vi "AlGaInPAs_v20c.vi"(2 "Debug Mode":bool, 3 "Elapsed Time(s)":dbl, 4 "State":enum16{"Edit", "Start", "Run", "End", "Idle"}(ring), 5 "Argument List In":string[](array[string])) -> (0 "Status Out":string, 1 "Argument List Out":string[](array[string]))   [LabVIEW 2011]
uses:
  high_level_proc/source_noDilute.ctl
  high_level_proc/source_noDilution.ctl
panel:
  in  "Array":refnum<vi>[](array[refnum])
  in  "Al bubbler":T1 caption="Al" {"Flow" format="%.2f"}
  in  "Se bubbler":T2={"Dilution"=FALSE, "Calculated"=0, "MFC1 flow"=0.0, "MFC2 flow"=10.0, "MFC3 flow"=100.0, "Bubbler (main)"={"Flow"=0.0, "Prep"=FALSE, "Run"=FALSE, "Active"=FALSE}} caption="Al" {"Bubbler (main)"."Flow" format="%.2f"; "MFC1 flow" format="%.4f"; "MFC3 flow" format="%.1f"; "MFC2 flow" format="%.2f"; "Calculated" items=["Flow", "MFC1", "MFC2", "MFC3"]}
  in  "P bubbler":T1 caption="Al" {"Flow" format="%.2f"}
  in  "As gas":T1 caption="Al" {"Flow" format="%.2f"}
  in  "P gas":T1 caption="Al" {"Flow" format="%.2f"}
  in  "In bubbler":T1 caption="Al" {"Flow" format="%.2f"}
  in  "Tab Control":T3(tab)
  out "Al Prep":bool caption="Pre-run"
  out "Al Run":bool caption="Run"
  out "Al Flow":dbl caption="Al Flow (0-100 sscm)" format="%.2f"
  out "Ga MFC1 flow":dbl caption="R1 (0-10 sscm)" format="%.4f"
  out "Ga MFC3 flow":dbl=100.0 caption="R3 (0-1000 sscm)" format="%.1f"
  out "Ga MFC2 flow":dbl=10.0 caption="R2 (0-100 sscm)" format="%.2f"
  out "Ga Calculated":u16(ring)=1 caption="Calculated" items=["Ga flow", "MFC1", "MFC2", "MFC3"]
  out "Ga Dilution":bool caption="Dilute"
  out "Ga Prep":bool caption="Pre-run"
  out "Ga Run":bool caption="Run"
  out "Ga Flow":dbl caption="Ga Flow (0-10 sscm)" format="%.2f"
  out "In Prep":bool caption="Pre-run"
  out "In Run":bool caption="Run"
  out "In Flow":dbl caption="In Flow (0-100 sscm)" format="%.2f"
  out "P gas Run":bool caption="Run"
  out "P gas Prep":bool caption="Pre-run"
  out "P gas Flow":dbl caption="PH3 Flow (0-100 sscm)" format="%.2f"
  out "As gas Prep":bool caption="Pre-run"
  out "As gas Run":bool caption="Run"
  out "As gas Flow":dbl caption="AsH3 Flow (0-10 sscm)" format="%.2f"
  out "P liq Prep":bool caption="Pre-run"
  out "P liq Run":bool caption="Run"
  out "P liq Flow":dbl caption="P bubbler Flow (0-100 sscm)" format="%.2f"
  out "Se MFC1 flow":dbl caption="R1 (0-10 sscm)" format="%.4f"
  out "Se MFC3 flow":dbl=100.0 caption="R3 (0-1000 sscm)" format="%.1f"
  out "Se MFC2 flow":dbl=10.0 caption="R2 (0-100 sscm)" format="%.2f"
  out "Se Calculated":u16(ring)=1 caption="Calculated" items=["Ga flow", "MFC1", "MFC2", "MFC3"]
  out "Se Dilution":bool caption="Dilute"
  out "Se Prep":bool caption="Pre-run"
  out "Se Run":bool caption="Run"
  out "Se Flow":dbl caption="Se Flow (0-10 sscm)" format="%.2f"
  in  "Ga bubbler":T2={"Dilution"=FALSE, "Calculated"=0, "MFC1 flow"=0.0, "MFC2 flow"=10.0, "MFC3 flow"=100.0, "Bubbler (main)"={"Flow"=0.0, "Prep"=FALSE, "Run"=FALSE, "Active"=FALSE}} caption="Al" {"Bubbler (main)"."Flow" format="%.2f"; "MFC1 flow" format="%.4f"; "MFC3 flow" format="%.1f"; "MFC2 flow" format="%.2f"; "Calculated" items=["Flow", "MFC1", "MFC2", "MFC3"]}
  out "prep_done":bool
  out "run started":bool
  out "first":bool=TRUE
  out "total time":dbl
  out "is OK?":bool
  in  "prep_time":dbl
  in  "Cancel":bool
  in  "OK":bool
  out "tTotal(s) 2":dbl
  # "s"
  # "Add pre-run time to run time in editor."
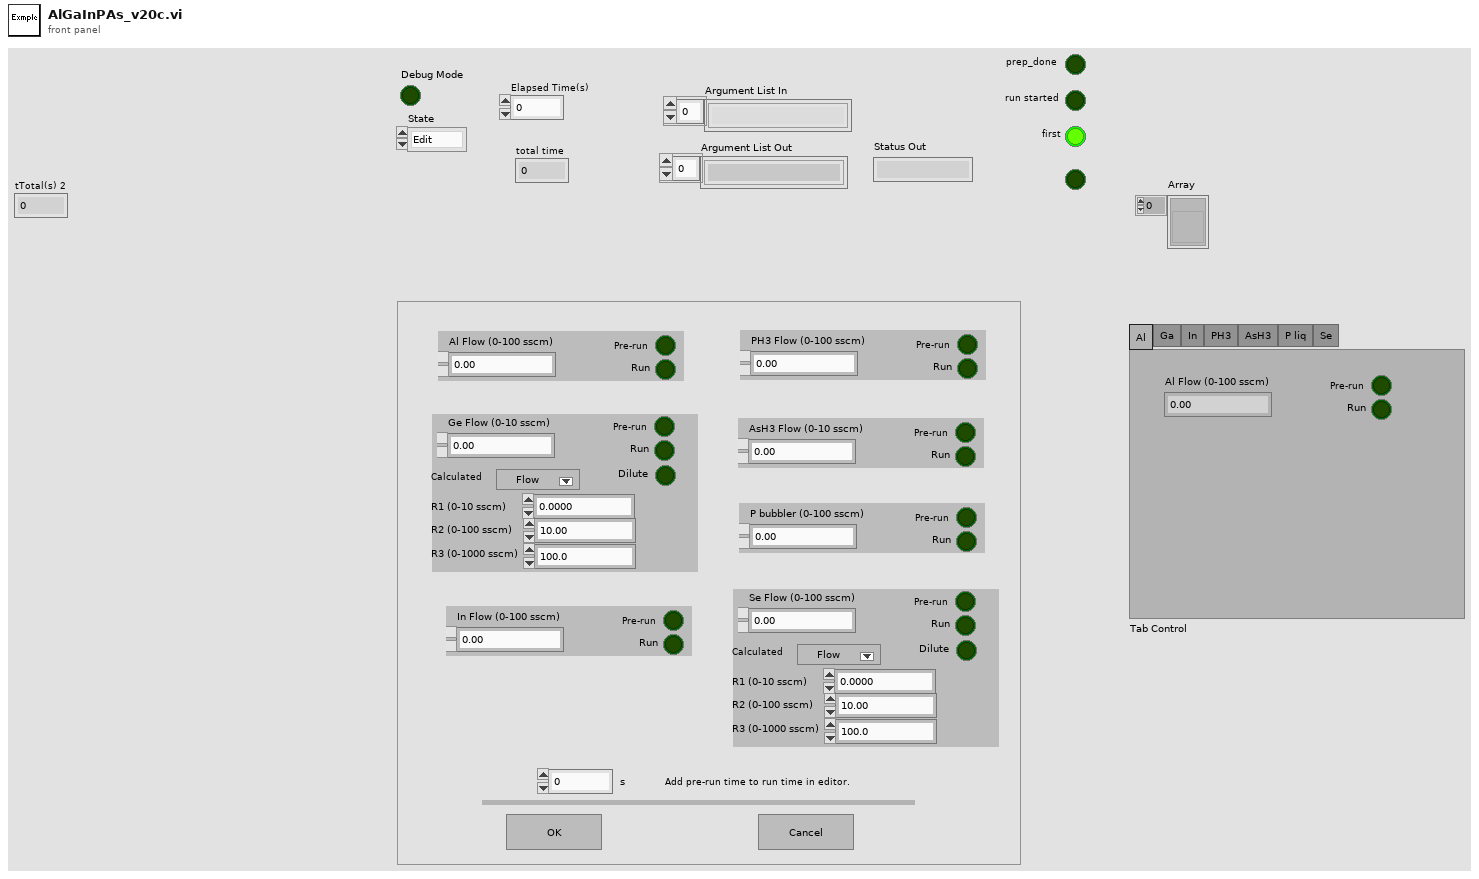
[diagram p1: front panel]
types:
  T1 = typedef "source_noDilution.ctl" = cluster{"Flow":dbl, "Prep":bool, "Run":bool, "Active":bool}
  T2 = typedef "source_noDilute.ctl" = cluster{"Dilution":bool, "Calculated":u16, "MFC1 flow":dbl, "MFC2 flow":dbl, "MFC3 flow":dbl, "Bubbler (main)":T1}
  T3 = enum32{"Al", "Ga", "In", "PH3", "AsH3", "P liq", "Se"}
  T4 = enum16{"Discrete", "Continuous", "Instantaneous", "Finite"}
  T5 = enum32{"Invalid", "Default", "Floating", "Floating/Auto-Hide", "Modal"}
  T6 = enum8{"Enabled", "Disabled", "Disabled and Grayed Out"}
  T7 = cluster{"Flow":dbl, "Prep":bool, "Run":bool, "Active":bool}
  T8 = cluster{"Dilution":bool, "Calculated":u16, "MFC1 flow":dbl, "MFC2 flow":dbl, "MFC3 flow":dbl, "Bubbler (main)":T1}
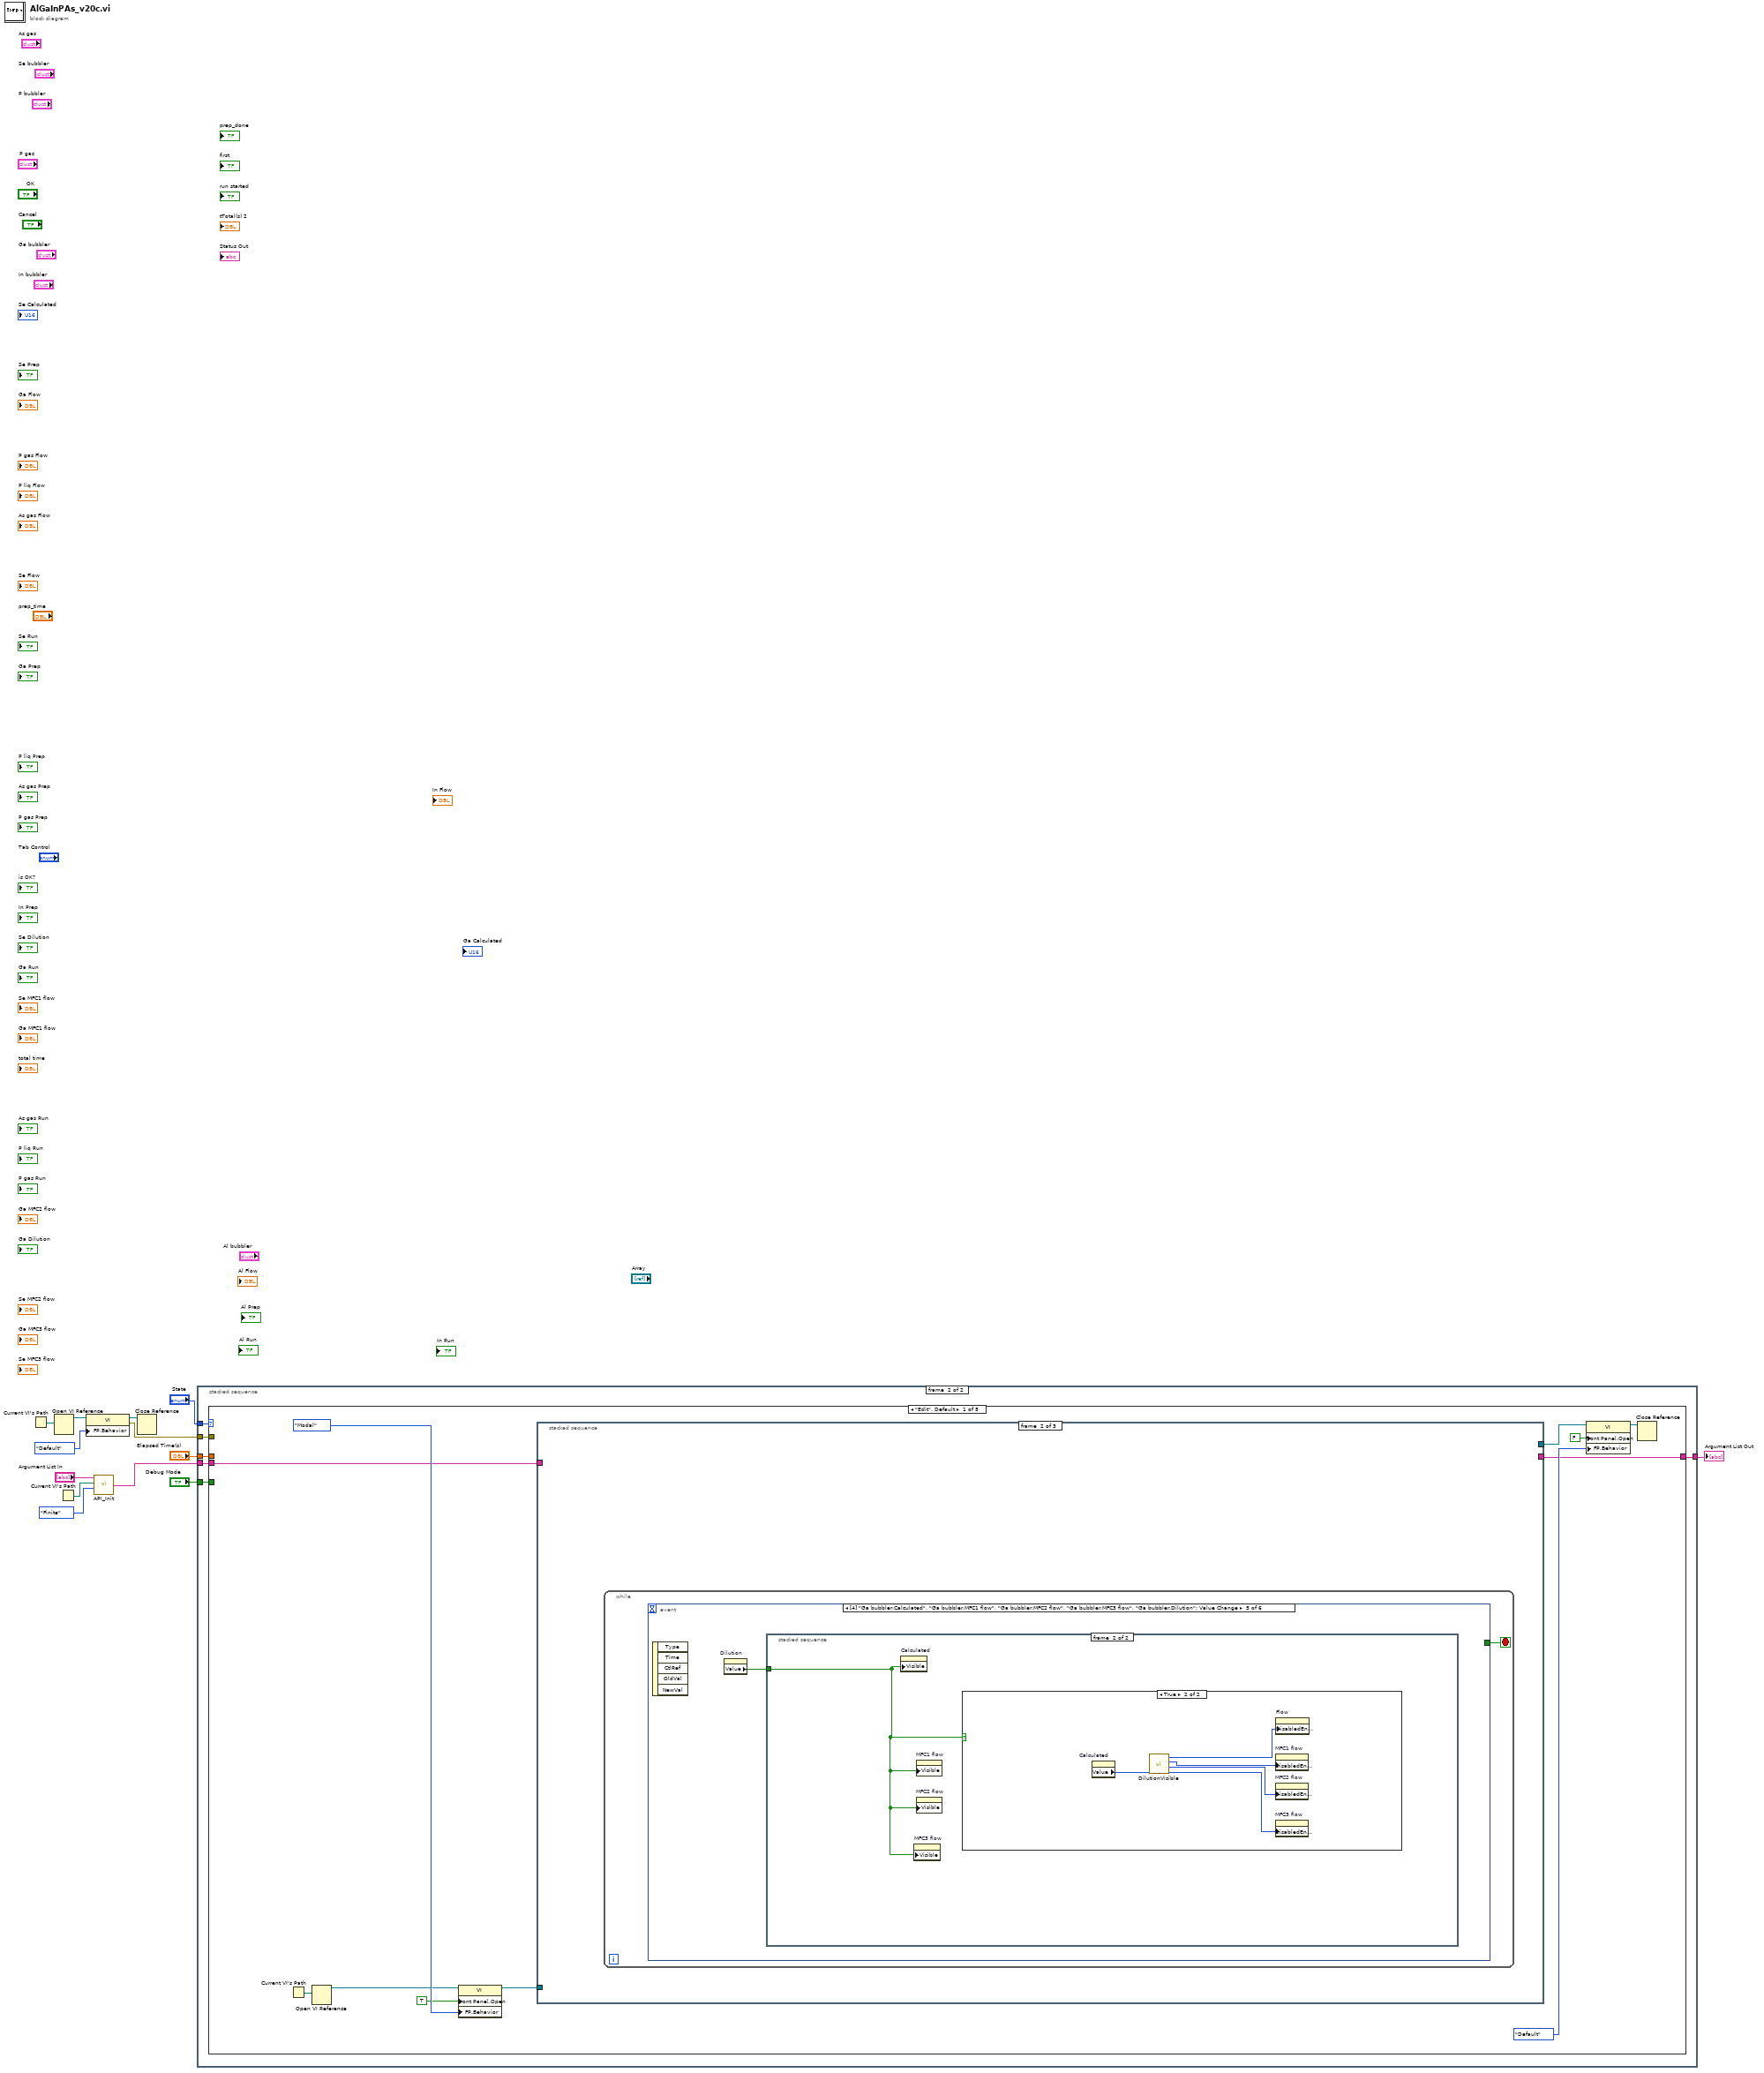
[diagram p0: block diagram]
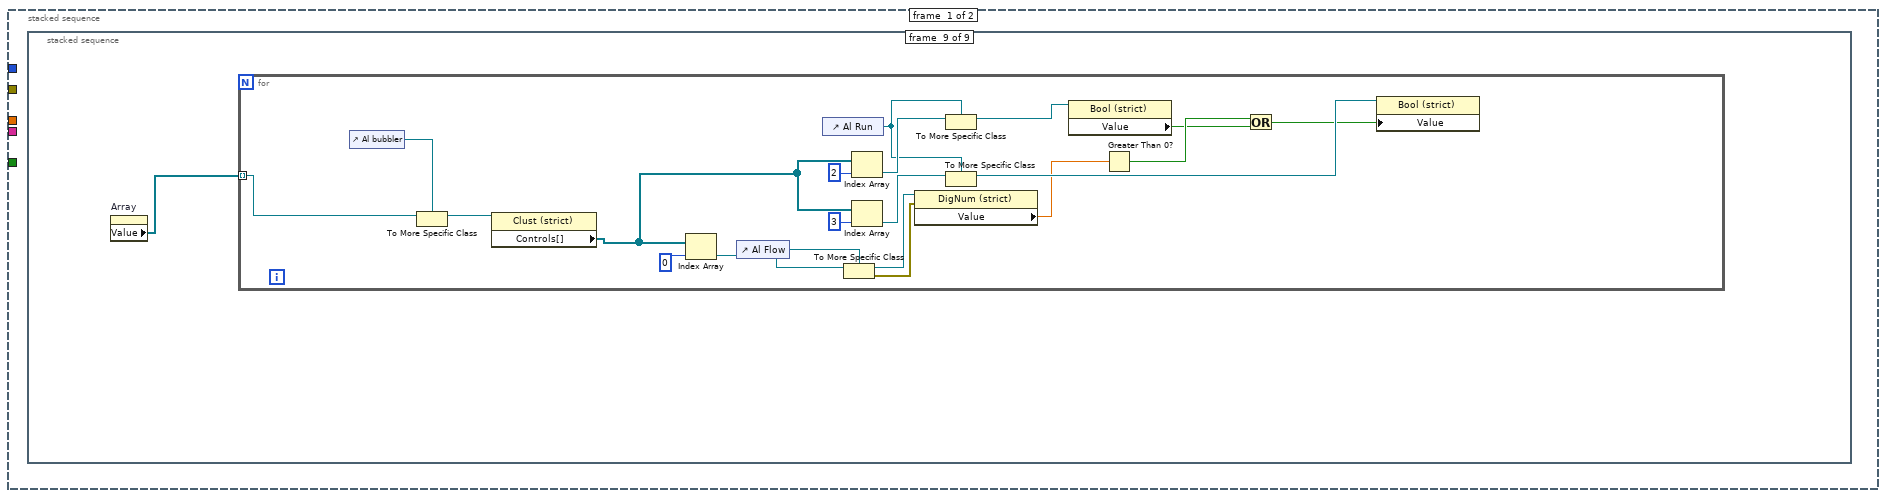
[diagram p2: hidden frame]
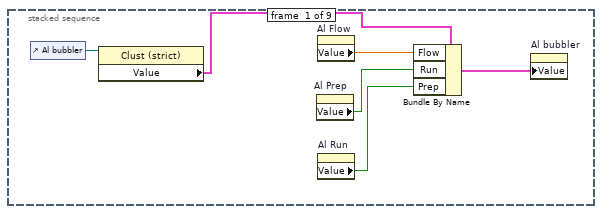
[diagram p3: hidden frame]
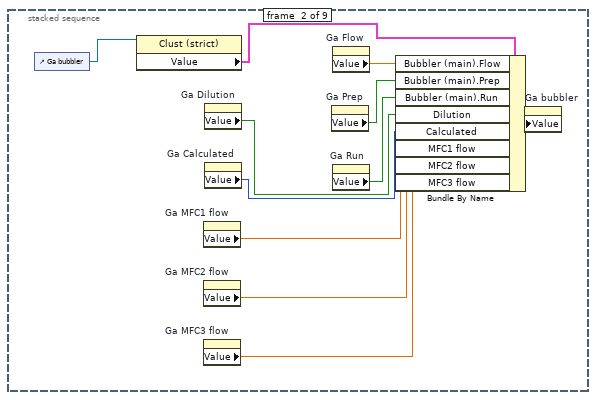
[diagram p4: hidden frame]
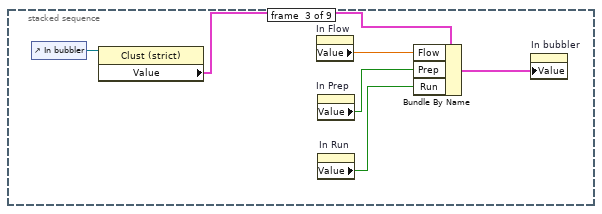
[diagram p5: hidden frame]
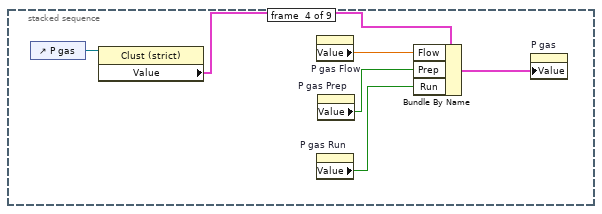
[diagram p6: hidden frame]
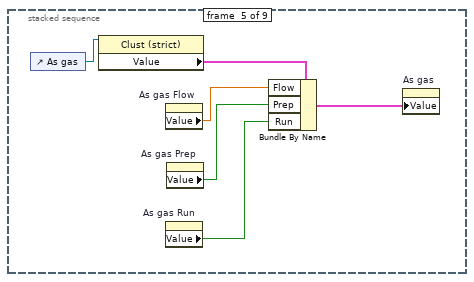
[diagram p7: hidden frame]
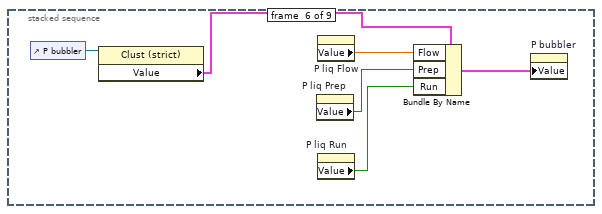
[diagram p8: hidden frame]
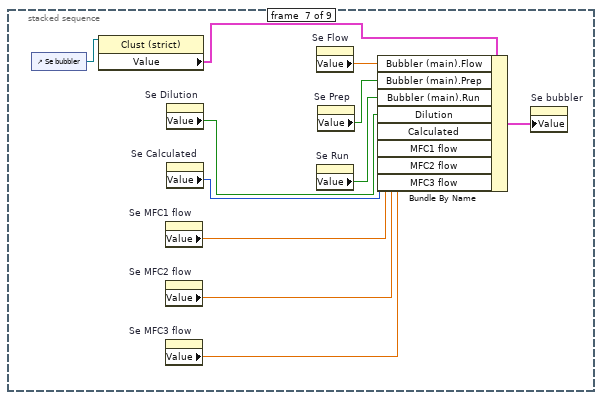
[diagram p9: hidden frame]
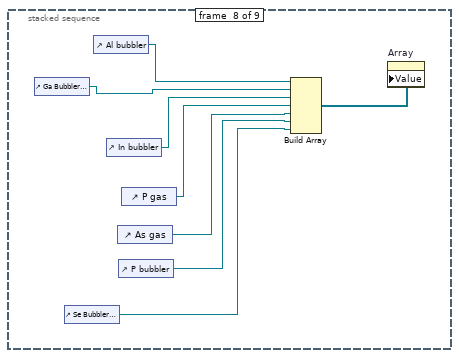
[diagram p10: hidden frame]
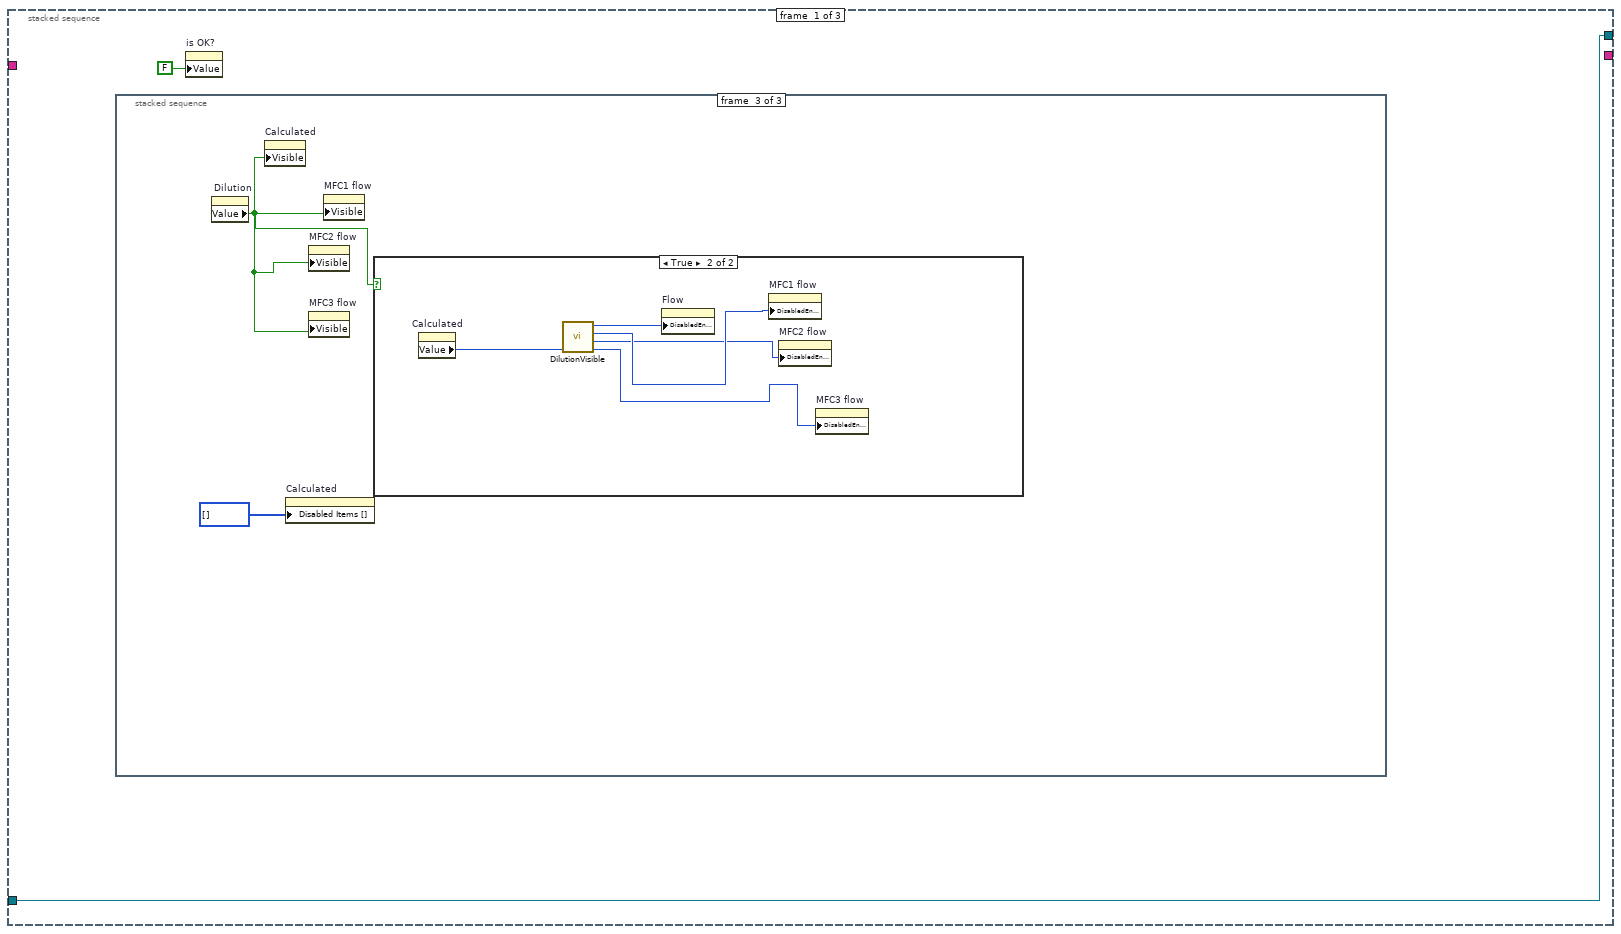
[diagram p11: hidden frame]
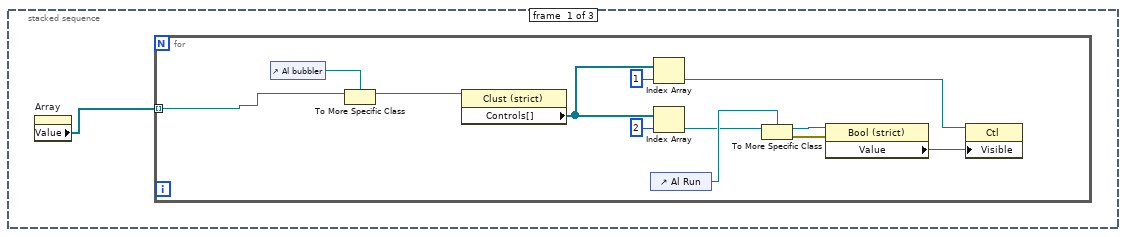
[diagram p12: hidden frame]
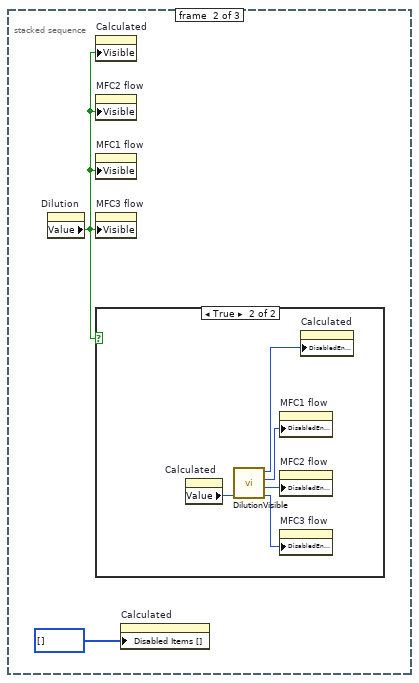
[diagram p13: hidden frame]
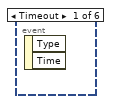
[diagram p16: hidden frame]
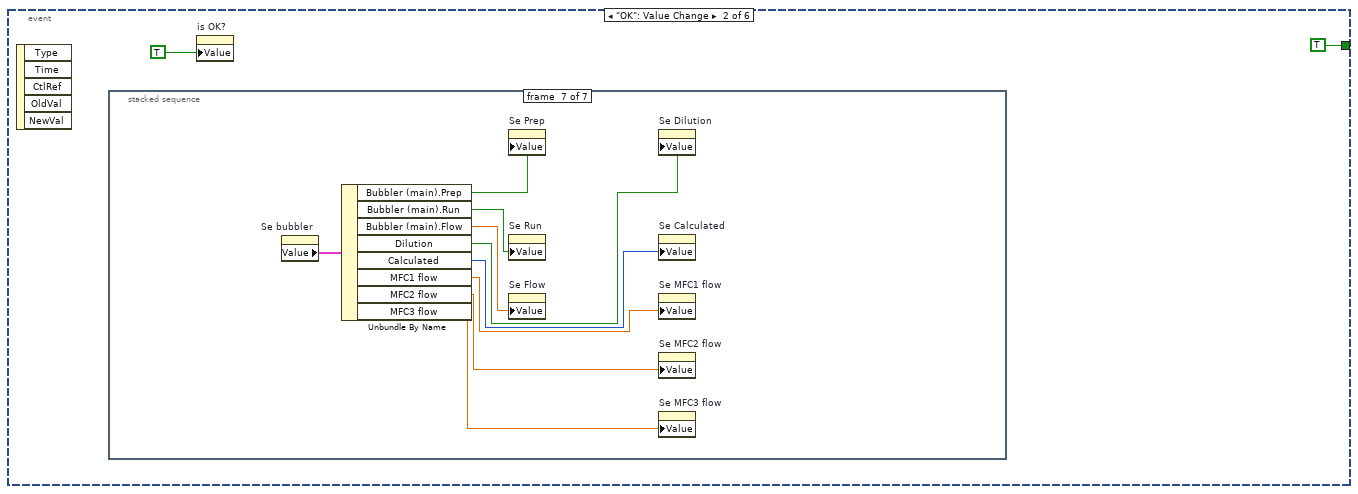
[diagram p17: hidden frame]
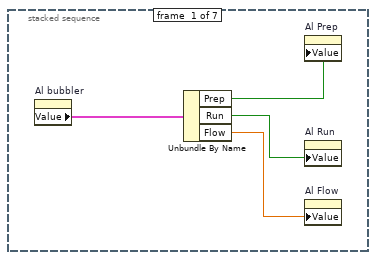
[diagram p18: hidden frame]
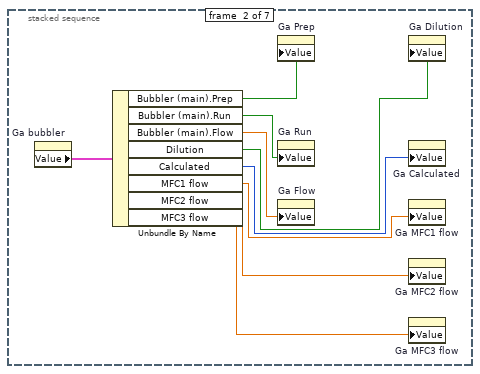
[diagram p19: hidden frame]
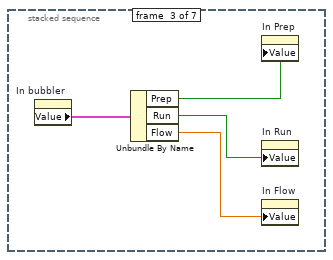
[diagram p20: hidden frame]
diagram:
  n1 = Current VI's Path() -> (path=w9:path)
  n2 = Open VI Reference(vi path=w9) -> (vi reference=w8:refnum<vi>)  [unwired: 1 in, 5 out]
  n3 = Current VI's Path() -> (path=w4:path)
  n4 = property class="VI"(reference=w8, "FP.Behavior"=T5."Default" ("Front Panel Window:Behavior")) -> (reference out=w6:refnum<vi>, error out=w5:errorcluster)  [unwired: 1 in]
  n5 = call "API_Init.vi"("API Mode"=T4."Finite", "VI Path"=w4, "Argument List In"="Argument List In") -> ("Argument List Out"=w1:string[])  [unwired: 1 in]
  n6 = Close Reference(reference=w6) -> ()  [unwired: 1 in, 1 out]
  n7 = stacked-sequence {
    tunnel: "State" -> [_ w100]
    tunnel: "Debug Mode" -> [_ w99]
    tunnel: "Elapsed Time(s)" -> [_ w98]
    tunnel: [_ w97] -> w10
    tunnel: w5 -> [_ w96]
    tunnel: w1 -> [_ w95]
    frame #0 {
      n8 = stacked-sequence {
        frame #0 {
          n9 = control-ref of="Al bubbler"() -> (w16:refnum<vi>)
          n10 = property class="Clust (strict)"(reference=w16) -> ("Value"=w15:T7)  [unwired: 1 in, 2 out]
          n11 = property on="Al Prep" class="Bool (strict)"() -> ("Value"=w18:bool)  [unwired: 2 in, 2 out]
          n12 = property on="Al Flow" class="DigNum (strict)"() -> ("Value"=w19:dbl)  [unwired: 2 in, 2 out]
          n13 = property on="Al Run" class="Bool (strict)"() -> ("Value"=w17:bool)  [unwired: 2 in, 2 out]
          n14 = Bundle By Name(cluster=w15, "Flow"=w19, "Run"=w18, "Prep"=w17) -> (w14:T7)
          n15 = property on="Al bubbler" class="Clust (strict)"("Value"=w14) -> ()  [unwired: 2 in, 2 out]
        }
        frame #1 {
          n16 = control-ref of="Ga bubbler"() -> (w20:refnum<vi>)
          n17 = property class="Clust (strict)"(reference=w20) -> ("Value"=w21:T8)  [unwired: 1 in, 2 out]
          n18 = property on="Ga MFC1 flow" class="DigNum (strict)"() -> ("Value"=w28:dbl)  [unwired: 2 in, 2 out]
          n19 = property on="Ga MFC2 flow" class="DigNum (strict)"() -> ("Value"=w29:dbl)  [unwired: 2 in, 2 out]
          n20 = property on="Ga MFC3 flow" class="DigNum (strict)"() -> ("Value"=w30:dbl)  [unwired: 2 in, 2 out]
          n21 = property on="Ga Dilution" class="Bool (strict)"() -> ("Value"=w27:bool)  [unwired: 2 in, 2 out]
          n22 = property on="Ga Calculated" class="Ring (strict)"() -> ("Value"=w25:u16)  [unwired: 2 in, 2 out]
          n23 = property on="Ga Prep" class="Bool (strict)"() -> ("Value"=w24:bool)  [unwired: 2 in, 2 out]
          n24 = property on="Ga Flow" class="DigNum (strict)"() -> ("Value"=w23:dbl)  [unwired: 2 in, 2 out]
          n25 = property on="Ga Run" class="Bool (strict)"() -> ("Value"=w26:bool)  [unwired: 2 in, 2 out]
          n26 = Bundle By Name(cluster=w21, "Bubbler (main).Flow"=w23, "Bubbler (main).Prep"=w24, "Bubbler (main).Run"=w26, "Dilution"=w27, "Calculated"=w25, "MFC1 flow"=w28, "MFC2 flow"=w29, "MFC3 flow"=w30) -> (w22:T8)
          n27 = property on="Ga bubbler" class="Clust (strict)"("Value"=w22) -> ()  [unwired: 2 in, 2 out]
        }
        frame #2 {
          n28 = control-ref of="In bubbler"() -> (w31:refnum<vi>)
          n29 = property class="Clust (strict)"(reference=w31) -> ("Value"=w32:T7)  [unwired: 1 in, 2 out]
          n30 = property on="In Flow" class="DigNum (strict)"() -> ("Value"=w33:dbl)  [unwired: 2 in, 2 out]
          n31 = property on="In Prep" class="Bool (strict)"() -> ("Value"=w35:bool)  [unwired: 2 in, 2 out]
          n32 = property on="In Run" class="Bool (strict)"() -> ("Value"=w36:bool)  [unwired: 2 in, 2 out]
          n33 = Bundle By Name(cluster=w32, "Flow"=w33, "Prep"=w35, "Run"=w36) -> (w34:T7)
          n34 = property on="In bubbler" class="Clust (strict)"("Value"=w34) -> ()  [unwired: 2 in, 2 out]
        }
        frame #3 {
          n35 = control-ref of="P gas"() -> (w37:refnum<vi>)
          n36 = property class="Clust (strict)"(reference=w37) -> ("Value"=w38:T7)  [unwired: 1 in, 2 out]
          n37 = property on="P gas Flow" class="DigNum (strict)"() -> ("Value"=w39:dbl)  [unwired: 2 in, 2 out]
          n38 = property on="P gas Run" class="Bool (strict)"() -> ("Value"=w42:bool)  [unwired: 2 in, 2 out]
          n39 = property on="P gas Prep" class="Bool (strict)"() -> ("Value"=w41:bool)  [unwired: 2 in, 2 out]
          n40 = Bundle By Name(cluster=w38, "Flow"=w39, "Prep"=w41, "Run"=w42) -> (w40:T7)
          n41 = property on="P gas" class="Clust (strict)"("Value"=w40) -> ()  [unwired: 2 in, 2 out]
        }
        frame #4 {
          n42 = control-ref of="As gas"() -> (w44:refnum<vi>)
          n43 = property class="Clust (strict)"(reference=w44) -> ("Value"=w43:T7)  [unwired: 1 in, 2 out]
          n44 = property on="As gas Flow" class="DigNum (strict)"() -> ("Value"=w46:dbl)  [unwired: 2 in, 2 out]
          n45 = property on="As gas Run" class="Bool (strict)"() -> ("Value"=w48:bool)  [unwired: 2 in, 2 out]
          n46 = property on="As gas Prep" class="Bool (strict)"() -> ("Value"=w47:bool)  [unwired: 2 in, 2 out]
          n47 = Bundle By Name(cluster=w43, "Flow"=w46, "Prep"=w47, "Run"=w48) -> (w45:T7)
          n48 = property on="As gas" class="Clust (strict)"("Value"=w45) -> ()  [unwired: 2 in, 2 out]
        }
        frame #5 {
          n49 = control-ref of="P bubbler"() -> (w49:refnum<vi>)
          n50 = property class="Clust (strict)"(reference=w49) -> ("Value"=w50:T7)  [unwired: 1 in, 2 out]
          n51 = property on="P liq Prep" class="Bool (strict)"() -> ("Value"=w53:bool)  [unwired: 2 in, 2 out]
          n52 = property on="P liq Flow" class="DigNum (strict)"() -> ("Value"=w52:dbl)  [unwired: 2 in, 2 out]
          n53 = property on="P liq Run" class="Bool (strict)"() -> ("Value"=w54:bool)  [unwired: 2 in, 2 out]
          n54 = Bundle By Name(cluster=w50, "Flow"=w52, "Prep"=w53, "Run"=w54) -> (w51:T7)
          n55 = property on="P bubbler" class="Clust (strict)"("Value"=w51) -> ()  [unwired: 2 in, 2 out]
        }
        frame #6 {
          n56 = control-ref of="Se bubbler"() -> (w55:refnum<vi>)
          n57 = property class="Clust (strict)"(reference=w55) -> ("Value"=w56:T8)  [unwired: 1 in, 2 out]
          n58 = property on="Se MFC1 flow" class="DigNum (strict)"() -> ("Value"=w63:dbl)  [unwired: 2 in, 2 out]
          n59 = property on="Se MFC2 flow" class="DigNum (strict)"() -> ("Value"=w64:dbl)  [unwired: 2 in, 2 out]
          n60 = property on="Se MFC3 flow" class="DigNum (strict)"() -> ("Value"=w65:dbl)  [unwired: 2 in, 2 out]
          n61 = property on="Se Dilution" class="Bool (strict)"() -> ("Value"=w61:bool)  [unwired: 2 in, 2 out]
          n62 = property on="Se Calculated" class="Ring (strict)"() -> ("Value"=w62:u16)  [unwired: 2 in, 2 out]
          n63 = property on="Se Flow" class="DigNum (strict)"() -> ("Value"=w58:dbl)  [unwired: 2 in, 2 out]
          n64 = property on="Se Run" class="Bool (strict)"() -> ("Value"=w60:bool)  [unwired: 2 in, 2 out]
          n65 = property on="Se Prep" class="Bool (strict)"() -> ("Value"=w59:bool)  [unwired: 2 in, 2 out]
          n66 = Bundle By Name(cluster=w56, "Bubbler (main).Flow"=w58, "Bubbler (main).Prep"=w59, "Bubbler (main).Run"=w60, "Dilution"=w61, "Calculated"=w62, "MFC1 flow"=w63, "MFC2 flow"=w64, "MFC3 flow"=w65) -> (w57:T8)
          n67 = property on="Se bubbler" class="Clust (strict)"("Value"=w57) -> ()  [unwired: 2 in, 2 out]
        }
        frame #7 {
          n68 = control-ref of="Ga Bubbler (main)"() -> (w67:refnum<vi>)
          n69 = control-ref of="Se Bubbler (main)"() -> (w66:refnum<vi>)
          n70 = control-ref of="Al bubbler"() -> (w72:refnum<vi>)
          n71 = control-ref of="In bubbler"() -> (w71:refnum<vi>)
          n72 = control-ref of="As gas"() -> (w69:refnum<vi>)
          n73 = control-ref of="P bubbler"() -> (w68:refnum<vi>)
          n74 = control-ref of="P gas"() -> (w70:refnum<vi>)
          n75 = Build Array(w72, w67, w71, w70, w69, w68, w66) -> (w73:refnum<vi>[])
          n76 = property on="Array" class="Arr (strict)"("Value"=w73) -> ()  [unwired: 2 in, 2 out]
        }
        frame #8 {
          n77 = property on="Array" class="Arr (strict)"() -> ("Value"=w74:refnum<vi>[])  [unwired: 2 in, 2 out]
          n78 = for {
            tunnel: w74 -> [w75] mode=indexing
            n79 = control-ref of="Al bubbler"() -> (w78:refnum<vi>)
            n80 = To More Specific Class(target class=w78, reference=w75) -> (specific class reference=w77:refnum<vi>)  [unwired: 1 in, 1 out]
            n81 = property class="Clust (strict)"(reference=w77) -> ("Controls[]"=w76:refnum<vi>[])  [unwired: 1 in, 2 out]
            n82 = Index Array(array=w76, index=0) -> (element=w90:refnum<vi>)
            n83 = control-ref of="Al Flow"() -> (w89:refnum<vi>)
            n84 = control-ref of="Al Run"() -> (w91:refnum<vi>)
            n85 = To More Specific Class(target class=w89, reference=w90) -> (specific class reference=w86:refnum<vi>, error out=w85:errorcluster)  [unwired: 1 in]
            n86 = Index Array(array=w76, index=2) -> (element=w93:refnum<vi>)
            n87 = Index Array(array=w76, index=3) -> (element=w92:refnum<vi>)
            n88 = property class="DigNum (strict)"(reference=w86, error in=w85) -> ("Value"=w84:dbl)  [unwired: 2 out]
            n89 = To More Specific Class(target class=w91, reference=w93) -> (specific class reference=w88:refnum<vi>)  [unwired: 1 in, 1 out]
            n90 = To More Specific Class(target class=w91, reference=w92) -> (specific class reference=w87:refnum<vi>)  [unwired: 1 in, 1 out]
            n91 = property class="Bool (strict)"(reference=w88) -> ("Value"=w83:bool)  [unwired: 1 in, 2 out]
            n92 = Greater Than 0?(x=w84) -> (x > 0?=w94:bool)
            n93 = Or(x=w94, y=w83) -> (x .or. y?=w82:bool)
            n94 = property class="Bool (strict)"(reference=w87, "Value"=w82) -> ()  [unwired: 1 in, 2 out]
          }
        }
      }
    }
    frame #1 {
      n95 = case shown="\"Edit\", Default" w100 {
        tunnel: w99 -> [_ w238 w256 _ _]
        tunnel: w98 -> [_ _ w257 _ _]
        tunnel: w95 -> [w102 w243 w255 w359 w360]
        tunnel: [w101 w242 w254 w359 w360] -> w97
        tunnel: w96 -> [_ _ _ _ _]
        frame "Edit", Default {
          n96 = Current VI's Path() -> (path=w107:path)
          n97 = Open VI Reference(vi path=w107) -> (vi reference=w106:refnum<vi>)  [unwired: 1 in, 5 out]
          n98 = property class="VI"(reference=w106, "Front Panel.Open"=TRUE ("Front Panel Window:Open"), "FP.Behavior"=T5."Modal" ("Front Panel Window:Behavior")) -> (reference out=w105:refnum<vi>)  [unwired: 1 in, 1 out]
          n99 = stacked-sequence {
            tunnel: w102 -> [_ _ w233]
            tunnel: w105 -> [w113 _ _]
            tunnel: [w113 _ _] -> w109
            tunnel: [_ _ w234] -> w101
            frame #0 {
              n100 = stacked-sequence {
                frame #0 {
                  n101 = property on="Array" class="Arr (strict)"() -> ("Value"=w114:refnum<vi>[])  [unwired: 2 in, 2 out]
                  n102 = for {
                    tunnel: w114 -> [w115] mode=indexing
                    n103 = control-ref of="Al bubbler"() -> (w116:refnum<vi>)
                    n104 = To More Specific Class(target class=w116, reference=w115) -> (specific class reference=w124:refnum<vi>)  [unwired: 1 in, 1 out]
                    n105 = property class="Clust (strict)"(reference=w124) -> ("Controls[]"=w123:refnum<vi>[])  [unwired: 1 in, 2 out]
                    n106 = control-ref of="Al Run"() -> (w121:refnum<vi>)
                    n107 = Index Array(array=w123, index=1) -> (element=w125:refnum<vi>)
                    n108 = Index Array(array=w123, index=2) -> (element=w120:refnum<vi>)
                    n109 = To More Specific Class(target class=w121, reference=w120) -> (specific class reference=w119:refnum<vi>, error out=w118:errorcluster)  [unwired: 1 in]
                    n110 = property class="Bool (strict)"(reference=w119, error in=w118) -> ("Value"=w117:bool)  [unwired: 2 out]
                    n111 = property class="Ctl"(reference=w125, "Visible"=w117) -> ()  [unwired: 1 in, 2 out]
                  }
                }
                frame #1 {
                  n112 = property on="Dilution" class="Bool (strict)"() -> ("Value"=w128:bool)  [unwired: 2 in, 2 out]
                  n113 = property on="Calculated" class="Ring (strict)"("Visible"=w128) -> ()  [unwired: 2 in, 2 out]
                  n114 = property on="MFC2 flow" class="DigNum (strict)"("Visible"=w128) -> ()  [unwired: 2 in, 2 out]
                  n115 = property on="MFC1 flow" class="DigNum (strict)"("Visible"=w128) -> ()  [unwired: 2 in, 2 out]
                  n116 = property on="MFC3 flow" class="DigNum (strict)"("Visible"=w128) -> ()  [unwired: 2 in, 2 out]
                  n117 = case shown="True" w128 {
                    frame False {
                    }
                    frame True {
                      n118 = property on="Calculated" class="Ring (strict)"() -> ("Value"=w130:u16)  [unwired: 2 in, 2 out]
                      n119 = call "DilutionVisible.vi"("calculated"=w130) -> ("MFC3"=w133:u16, "MFC2"=w132:u16, "MFC1"=w131:u16, "flow"=w129:u16)  [unwired: 3 in]
                      n120 = property on="MFC1 flow" class="DigNum (strict)"("DisabledEnum"=w131) -> ()  [unwired: 2 in, 2 out]
                      n121 = property on="MFC2 flow" class="DigNum (strict)"("DisabledEnum"=w132) -> ()  [unwired: 2 in, 2 out]
                      n122 = property on="MFC3 flow" class="DigNum (strict)"("DisabledEnum"=w133) -> ()  [unwired: 2 in, 2 out]
                      n123 = property on="Calculated" class="Ring (strict)"("DisabledEnum"=w129) -> ()  [unwired: 2 in, 2 out]
                    }
                  }
                  n124 = property on="Calculated" class="Ring (strict)"("Disabled Items []"=i32[] []) -> ()  [unwired: 2 in, 2 out]
                }
                frame #2 {
                  n125 = property on="Dilution" class="Bool (strict)"() -> ("Value"=w134:bool)  [unwired: 2 in, 2 out]
                  n126 = property on="Calculated" class="Ring (strict)"("Visible"=w134) -> ()  [unwired: 2 in, 2 out]
                  n127 = property on="Calculated" class="Ring (strict)"("Disabled Items []"=i32[] []) -> ()  [unwired: 2 in, 2 out]
                  n128 = property on="MFC2 flow" class="DigNum (strict)"("Visible"=w134) -> ()  [unwired: 2 in, 2 out]
                  n129 = property on="MFC3 flow" class="DigNum (strict)"("Visible"=w134) -> ()  [unwired: 2 in, 2 out]
                  n130 = property on="MFC1 flow" class="DigNum (strict)"("Visible"=w134) -> ()  [unwired: 2 in, 2 out]
                  n131 = case shown="True" w134 {
                    frame False {
                    }
                    frame True {
                      n132 = property on="Calculated" class="Ring (strict)"() -> ("Value"=w139:u16)  [unwired: 2 in, 2 out]
                      n133 = call "DilutionVisible.vi"("calculated"=w139) -> ("MFC3"=w137:u16, "MFC2"=w136:u16, "MFC1"=w138:u16, "flow"=w140:u16)  [unwired: 3 in]
                      n134 = property on="Flow" class="DigNum (strict)"("DisabledEnum"=w140) -> ()  [unwired: 2 in, 2 out]
                      n135 = property on="MFC1 flow" class="DigNum (strict)"("DisabledEnum"=w138) -> ()  [unwired: 2 in, 2 out]
                      n136 = property on="MFC2 flow" class="DigNum (strict)"("DisabledEnum"=w136) -> ()  [unwired: 2 in, 2 out]
                      n137 = property on="MFC3 flow" class="DigNum (strict)"("DisabledEnum"=w137) -> ()  [unwired: 2 in, 2 out]
                    }
                  }
                }
              }
              n138 = property on="is OK?" class="Bool (strict)"("Value"=FALSE ("is OK?")) -> ()  [unwired: 2 in, 2 out]
            }
            frame #1 {
              n139 = while {
                stop <- w141 stop-if-true
                n140 = event shown="[4] \"Ga bubbler.Calculated\", \"Ga bubbler.MFC1 flow\", \"Ga bubbler.MFC2 flow\", \"Ga bubbler.MFC3 flow\", \"Ga bubbler.Dilution\": Value Change" {
                  selector: _ -> [_ _ _ _ _ _]
                  dyn-events: _ -> [_ _ _ _ _ _]
                  timeout: _ -> [_ _ _ _ _ _]
                  tunnel: [_ TRUE _ TRUE _ _] -> w141
                  event Timeout {
                    n141 = event-data() -> ()  [unwired: 1 in, 2 out]
                  }
                  event "OK": Value Change {
                    n142 = event-data() -> ()  [unwired: 1 in, 5 out]
                    n143 = stacked-sequence {
                      frame #0 {
                        n144 = property on="Al bubbler" class="Clust (strict)"() -> ("Value"=w144:T7)  [unwired: 2 in, 2 out]
                        n145 = Unbundle By Name(w144) -> ("Prep"=w147:bool, "Run"=w146:bool, "Flow"=w145:dbl)
                        n146 = property on="Al Prep" class="Bool (strict)"("Value"=w147) -> ()  [unwired: 2 in, 2 out]
                        n147 = property on="Al Run" class="Bool (strict)"("Value"=w146) -> ()  [unwired: 2 in, 2 out]
                        n148 = property on="Al Flow" class="DigNum (strict)"("Value"=w145) -> ()  [unwired: 2 in, 2 out]
                      }
                      frame #1 {
                        n149 = property on="Ga bubbler" class="Clust (strict)"() -> ("Value"=w156:T8)  [unwired: 2 in, 2 out]
                        n150 = Unbundle By Name(w156) -> ("Bubbler (main).Prep"=w155:bool, "Bubbler (main).Run"=w154:bool, "Bubbler (main).Flow"=w153:dbl, "Dilution"=w152:bool, "Calculated"=w151:u16, "MFC1 flow"=w150:dbl, "MFC2 flow"=w149:dbl, "MFC3 flow"=w148:dbl)
                        n151 = property on="Ga Prep" class="Bool (strict)"("Value"=w155) -> ()  [unwired: 2 in, 2 out]
                        n152 = property on="Ga Run" class="Bool (strict)"("Value"=w154) -> ()  [unwired: 2 in, 2 out]
                        n153 = property on="Ga Flow" class="DigNum (strict)"("Value"=w153) -> ()  [unwired: 2 in, 2 out]
                        n154 = property on="Ga Dilution" class="Bool (strict)"("Value"=w152) -> ()  [unwired: 2 in, 2 out]
                        n155 = property on="Ga Calculated" class="Ring (strict)"("Value"=w151) -> ()  [unwired: 2 in, 2 out]
                        n156 = property on="Ga MFC1 flow" class="DigNum (strict)"("Value"=w150) -> ()  [unwired: 2 in, 2 out]
                        n157 = property on="Ga MFC2 flow" class="DigNum (strict)"("Value"=w149) -> ()  [unwired: 2 in, 2 out]
                        n158 = property on="Ga MFC3 flow" class="DigNum (strict)"("Value"=w148) -> ()  [unwired: 2 in, 2 out]
                      }
                      frame #2 {
                        n159 = property on="In bubbler" class="Clust (strict)"() -> ("Value"=w160:T7)  [unwired: 2 in, 2 out]
                        n160 = Unbundle By Name(w160) -> ("Prep"=w159:bool, "Run"=w158:bool, "Flow"=w157:dbl)
                        n161 = property on="In Prep" class="Bool (strict)"("Value"=w159) -> ()  [unwired: 2 in, 2 out]
                        n162 = property on="In Run" class="Bool (strict)"("Value"=w158) -> ()  [unwired: 2 in, 2 out]
                        n163 = property on="In Flow" class="DigNum (strict)"("Value"=w157) -> ()  [unwired: 2 in, 2 out]
                      }
                      frame #3 {
                        n164 = property on="P gas" class="Clust (strict)"() -> ("Value"=w164:T7)  [unwired: 2 in, 2 out]
                        n165 = Unbundle By Name(w164) -> ("Prep"=w163:bool, "Run"=w162:bool, "Flow"=w161:dbl)
                        n166 = property on="P gas Prep" class="Bool (strict)"("Value"=w163) -> ()  [unwired: 2 in, 2 out]
                        n167 = property on="P gas Run" class="Bool (strict)"("Value"=w162) -> ()  [unwired: 2 in, 2 out]
                        n168 = property on="P gas Flow" class="DigNum (strict)"("Value"=w161) -> ()  [unwired: 2 in, 2 out]
                      }
                      frame #4 {
                        n169 = property on="As gas" class="Clust (strict)"() -> ("Value"=w168:T7)  [unwired: 2 in, 2 out]
                        n170 = Unbundle By Name(w168) -> ("Prep"=w167:bool, "Run"=w166:bool, "Flow"=w165:dbl)
                        n171 = property on="As gas Prep" class="Bool (strict)"("Value"=w167) -> ()  [unwired: 2 in, 2 out]
                        n172 = property on="As gas Run" class="Bool (strict)"("Value"=w166) -> ()  [unwired: 2 in, 2 out]
                        n173 = property on="As gas Flow" class="DigNum (strict)"("Value"=w165) -> ()  [unwired: 2 in, 2 out]
                      }
                      frame #5 {
                        n174 = property on="P bubbler" class="Clust (strict)"() -> ("Value"=w172:T7)  [unwired: 2 in, 2 out]
                        n175 = Unbundle By Name(w172) -> ("Prep"=w171:bool, "Run"=w170:bool, "Flow"=w169:dbl)
                        n176 = property on="P liq Prep" class="Bool (strict)"("Value"=w171) -> ()  [unwired: 2 in, 2 out]
                        n177 = property on="P liq Run" class="Bool (strict)"("Value"=w170) -> ()  [unwired: 2 in, 2 out]
                        n178 = property on="P liq Flow" class="DigNum (strict)"("Value"=w169) -> ()  [unwired: 2 in, 2 out]
                      }
                      frame #6 {
                        n179 = property on="Se bubbler" class="Clust (strict)"() -> ("Value"=w181:T8)  [unwired: 2 in, 2 out]
                        n180 = Unbundle By Name(w181) -> ("Bubbler (main).Prep"=w180:bool, "Bubbler (main).Run"=w179:bool, "Bubbler (main).Flow"=w178:dbl, "Dilution"=w177:bool, "Calculated"=w176:u16, "MFC1 flow"=w175:dbl, "MFC2 flow"=w174:dbl, "MFC3 flow"=w173:dbl)
                        n181 = property on="Se Prep" class="Bool (strict)"("Value"=w180) -> ()  [unwired: 2 in, 2 out]
                        n182 = property on="Se Run" class="Bool (strict)"("Value"=w179) -> ()  [unwired: 2 in, 2 out]
                        n183 = property on="Se Flow" class="DigNum (strict)"("Value"=w178) -> ()  [unwired: 2 in, 2 out]
                        n184 = property on="Se Dilution" class="Bool (strict)"("Value"=w177) -> ()  [unwired: 2 in, 2 out]
                        n185 = property on="Se Calculated" class="Ring (strict)"("Value"=w176) -> ()  [unwired: 2 in, 2 out]
                        n186 = property on="Se MFC1 flow" class="DigNum (strict)"("Value"=w175) -> ()  [unwired: 2 in, 2 out]
                        n187 = property on="Se MFC2 flow" class="DigNum (strict)"("Value"=w174) -> ()  [unwired: 2 in, 2 out]
                        n188 = property on="Se MFC3 flow" class="DigNum (strict)"("Value"=w173) -> ()  [unwired: 2 in, 2 out]
                      }
                    }
                    n189 = property on="is OK?" class="Bool (strict)"("Value"=TRUE ("is OK?")) -> ()  [unwired: 2 in, 2 out]
                  }
                  event Value Change {
                    n190 = event-data() -> ()  [unwired: 1 in, 5 out]
                    n191 = property on="Array" class="Arr (strict)"() -> ("Value"=w182:refnum<vi>[])  [unwired: 2 in, 2 out]
                    n192 = for {
                      tunnel: w182 -> [w184] mode=indexing
                      n193 = control-ref of="Al bubbler"() -> (w183:refnum<vi>)
                      n194 = To More Specific Class(target class=w183, reference=w184) -> (specific class reference=w192:refnum<vi>)  [unwired: 1 in, 1 out]
                      n195 = property class="Clust (strict)"(reference=w192) -> ("Controls[]"=w191:refnum<vi>[])  [unwired: 1 in, 2 out]
                      n196 = control-ref of="Al Run"() -> (w185:refnum<vi>)
                      n197 = Index Array(array=w191, index=1) -> (element=w193:refnum<vi>)
                      n198 = Index Array(array=w191, index=2) -> (element=w189:refnum<vi>)
                      n199 = To More Specific Class(target class=w185, reference=w189) -> (specific class reference=w188:refnum<vi>, error out=w187:errorcluster)  [unwired: 1 in]
                      n200 = property class="Bool (strict)"(reference=w188, error in=w187) -> ("Value"=w186:bool)  [unwired: 2 out]
                      n201 = property class="Ctl"(reference=w193, "Visible"=w186) -> ()  [unwired: 1 in, 2 out]
                    }
                  }
                  event "Cancel": Value Change {
                    n202 = event-data() -> ()  [unwired: 1 in, 5 out]
                  }
                  event Value Change {
                    n203 = event-data() -> ()  [unwired: 1 in, 5 out]
                    n204 = property on="Dilution" class="Bool (strict)"() -> ("Value"=w196:bool)  [unwired: 2 in, 2 out]
                    n205 = stacked-sequence {
                      tunnel: w196 -> [w197 w207]
                      frame #0 {
                        n206 = case shown="True" w197 {
                          frame False {
                          }
                          frame True {
                            n207 = property on="MFC1 flow" class="DigNum (strict)"() -> ("Value"=w205:dbl)  [unwired: 2 in, 2 out]
                            n208 = property on="MFC2 flow" class="DigNum (strict)"() -> ("Value"=w204:dbl)  [unwired: 2 in, 2 out]
                            n209 = property on="MFC3 flow" class="DigNum (strict)"() -> ("Value"=w203:dbl)  [unwired: 2 in, 2 out]
                            n210 = property on="Flow" class="DigNum (strict)"() -> ("Value"=w199:dbl)  [unwired: 2 in, 2 out]
                            n211 = property on="Calculated" class="Ring (strict)"() -> ("Value"=w206:u16)  [unwired: 2 in, 2 out]
                            n212 = call "dilutionCalc.vi"("Calculated"=w206, "MFC3"=w203, "MFC2"=w204, "MFC1"=w205, "flow"=w199) -> ("MFC3 out"=w200:dbl, "MFC2 out"=w201:dbl, "MFC1 out"=w202:dbl, "flow out"=w198:dbl)  [unwired: 1 in]
                            n213 = property on="Flow" class="DigNum (strict)"("Value"=w198) -> ()  [unwired: 2 in, 2 out]
                            n214 = property on="MFC1 flow" class="DigNum (strict)"("Value"=w202) -> ()  [unwired: 2 in, 2 out]
                            n215 = property on="MFC2 flow" class="DigNum (strict)"("Value"=w201) -> ()  [unwired: 2 in, 2 out]
                            n216 = property on="MFC3 flow" class="DigNum (strict)"("Value"=w200) -> ()  [unwired: 2 in, 2 out]
                          }
                        }
                      }
                      frame #1 {
                        n217 = property on="Calculated" class="Ring (strict)"("Visible"=w207) -> ()  [unwired: 2 in, 2 out]
                        n218 = property on="MFC3 flow" class="DigNum (strict)"("Visible"=w207) -> ()  [unwired: 2 in, 2 out]
                        n219 = property on="MFC1 flow" class="DigNum (strict)"("Visible"=w207) -> ()  [unwired: 2 in, 2 out]
                        n220 = property on="MFC2 flow" class="DigNum (strict)"("Visible"=w207) -> ()  [unwired: 2 in, 2 out]
                        n221 = case shown="True" w207 {
                          frame False {
                            n222 = property on="Calculated" class="Ring (strict)"("DisabledEnum"=T6."Enabled" ("Disabled")) -> ()  [unwired: 2 in, 2 out]
                          }
                          frame True {
                            n223 = property on="Calculated" class="Ring (strict)"() -> ("Value"=w210:u16)  [unwired: 2 in, 2 out]
                            n224 = call "DilutionVisible.vi"("calculated"=w210) -> ("MFC3"=w213:u16, "MFC2"=w212:u16, "MFC1"=w211:u16, "flow"=w209:u16)  [unwired: 3 in]
                            n225 = property on="MFC1 flow" class="DigNum (strict)"("DisabledEnum"=w211) -> ()  [unwired: 2 in, 2 out]
                            n226 = property on="MFC2 flow" class="DigNum (strict)"("DisabledEnum"=w212) -> ()  [unwired: 2 in, 2 out]
                            n227 = property on="MFC3 flow" class="DigNum (strict)"("DisabledEnum"=w213) -> ()  [unwired: 2 in, 2 out]
                            n228 = property on="Flow" class="DigNum (strict)"("DisabledEnum"=w209) -> ()  [unwired: 2 in, 2 out]
                          }
                        }
                      }
                    }
                  }
                  event Value Change {
                    n229 = event-data() -> ()  [unwired: 1 in, 5 out]
                    n230 = property on="Dilution" class="Bool (strict)"() -> ("Value"=w214:bool)  [unwired: 2 in, 2 out]
                    n231 = stacked-sequence {
                      tunnel: w214 -> [w215 w225]
                      frame #0 {
                        n232 = case shown="False" w215 {
                          frame False {
                          }
                          frame True {
                            n233 = property on="MFC3 flow" class="DigNum (strict)"() -> ("Value"=w219:dbl)  [unwired: 2 in, 2 out]
                            n234 = property on="MFC2 flow" class="DigNum (strict)"() -> ("Value"=w220:dbl)  [unwired: 2 in, 2 out]
                            n235 = property on="MFC1 flow" class="DigNum (strict)"() -> ("Value"=w221:dbl)  [unwired: 2 in, 2 out]
                            n236 = property on="Flow" class="DigNum (strict)"() -> ("Value"=w223:dbl)  [unwired: 2 in, 2 out]
                            n237 = property on="Calculated" class="Ring (strict)"() -> ("Value"=w224:u16)  [unwired: 2 in, 2 out]
                            n238 = call "dilutionCalc.vi"("Calculated"=w224, "MFC3"=w219, "MFC2"=w220, "MFC1"=w221, "flow"=w223) -> ("MFC3 out"=w216:dbl, "MFC2 out"=w217:dbl, "MFC1 out"=w218:dbl, "flow out"=w222:dbl)  [unwired: 1 in]
                            n239 = property on="Flow" class="DigNum (strict)"("Value"=w222) -> ()  [unwired: 2 in, 2 out]
                            n240 = property on="MFC1 flow" class="DigNum (strict)"("Value"=w218) -> ()  [unwired: 2 in, 2 out]
                            n241 = property on="MFC2 flow" class="DigNum (strict)"("Value"=w217) -> ()  [unwired: 2 in, 2 out]
                            n242 = property on="MFC3 flow" class="DigNum (strict)"("Value"=w216) -> ()  [unwired: 2 in, 2 out]
                          }
                        }
                      }
                      frame #1 {
                        n243 = property on="Calculated" class="Ring (strict)"("Visible"=w225) -> ()  [unwired: 2 in, 2 out]
                        n244 = property on="MFC1 flow" class="DigNum (strict)"("Visible"=w225) -> ()  [unwired: 2 in, 2 out]
                        n245 = property on="MFC2 flow" class="DigNum (strict)"("Visible"=w225) -> ()  [unwired: 2 in, 2 out]
                        n246 = property on="MFC3 flow" class="DigNum (strict)"("Visible"=w225) -> ()  [unwired: 2 in, 2 out]
                        n247 = case shown="False" w225 {
                          frame False {
                            n248 = property on="Flow" class="DigNum (strict)"("DisabledEnum"=T6."Enabled" ("Disabled")) -> ()  [unwired: 2 in, 2 out]
                          }
                          frame True {
                            n249 = property on="Calculated" class="Ring (strict)"() -> ("Value"=w230:u16)  [unwired: 2 in, 2 out]
                            n250 = call "DilutionVisible.vi"("calculated"=w230) -> ("MFC3"=w227:u16, "MFC2"=w228:u16, "MFC1"=w229:u16, "flow"=w231:u16)  [unwired: 3 in]
                            n251 = property on="Flow" class="DigNum (strict)"("DisabledEnum"=w231) -> ()  [unwired: 2 in, 2 out]
                            n252 = property on="MFC2 flow" class="DigNum (strict)"("DisabledEnum"=w228) -> ()  [unwired: 2 in, 2 out]
                            n253 = property on="MFC1 flow" class="DigNum (strict)"("DisabledEnum"=w229) -> ()  [unwired: 2 in, 2 out]
                            n254 = property on="MFC3 flow" class="DigNum (strict)"("DisabledEnum"=w227) -> ()  [unwired: 2 in, 2 out]
                          }
                        }
                      }
                    }
                  }
                }
              }
            }
            frame #2 {
              n255 = property on="is OK?" class="Bool (strict)"() -> ("Value"=w232:bool)  [unwired: 2 in, 2 out]
              n256 = Not(x=w232) -> (.not. x?=w236:bool)
              n257 = Current VI's Path() -> (path=w235:path)
              n258 = call "API_Edit.vi"("Cancel"=w236, "OK"=w232, "VI Path"=w235, "Argument List In"=w233) -> ("Argument List Out"=w234:string[])
            }
          }
          n259 = property class="VI"(reference=w109, "Front Panel.Open"=FALSE ("Front Panel Window:Open"), "FP.Behavior"=T5."Default" ("Front Panel Window:Behavior")) -> (reference out=w110:refnum<vi>)  [unwired: 1 in, 1 out]
          n260 = Close Reference(reference=w110) -> ()  [unwired: 1 in, 1 out]
        }
        frame "Start" {
          n261 = property on="prep_time" class="DigNum (strict)"() -> ("Value"=w241:dbl)  [unwired: 2 in, 2 out]
          n262 = Greater Than 0?(x=w241) -> (x > 0?=w240:bool)
          n263 = Not(x=w238) -> (.not. x?=w237:bool)
          n264 = And(x=w237, y=w240) -> (x .and. y?=w239:bool)
          n265 = case shown="True" w239 {
            frame False {
            }
            frame True {
              n266 = property on="Ga bubbler" class="Clust (strict)"() -> ("Value"=w251:T8)  [unwired: 2 in, 2 out]
              n267 = property on="P gas" class="Clust (strict)"() -> ("Value"=w249:T7)  [unwired: 2 in, 2 out]
              n268 = property on="Al bubbler" class="Clust (strict)"() -> ("Value"=w252:T7)  [unwired: 2 in, 2 out]
              n269 = property on="In bubbler" class="Clust (strict)"() -> ("Value"=w250:T7)  [unwired: 2 in, 2 out]
              n270 = property on="Se bubbler" class="Clust (strict)"() -> ("Value"=w246:T8)  [unwired: 2 in, 2 out]
              n271 = property on="As gas" class="Clust (strict)"() -> ("Value"=w248:T7)  [unwired: 2 in, 2 out]
              n272 = property on="P bubbler" class="Clust (strict)"() -> ("Value"=w247:T7)  [unwired: 2 in, 2 out]
              n273 = call "Set_V_III.vi"("Se bubbler"=w246, "P bubbler"=w247, "As gas"=w248, "P gas"=w249, "Run Started"=FALSE, "In bubbler"=w250, "Ga bubbler"=w251, "Al bubbler"=w252) -> ()  [unwired: 4 in]
            }
          }
          n274 = call "Set_Argument.vi"("Enable"=FALSE, "Argument"="run_started", "Argument List In"=w243) -> ("Argument List Out"=w242:string[])
        }
        frame "Run" {
          n275 = stacked-sequence {
            tunnel: w257 -> [_ w262 _ _]
            tunnel: w255 -> [w259 _ _ w336]
            tunnel: w256 -> [_ _ _ w334]
            tunnel: [_ _ _ w335] -> w254
            frame #0 {
              n276 = call "Get_Argument.vi"("Argument"="run_started", "Argument List"=w259) -> ("Enabled"=w258:bool)
              n277 = local write "run started"(w258) -> ()
            }
            frame #1 {
              n278 = property on="prep_time" class="DigNum (strict)"() -> ("Value"=w263:dbl)  [unwired: 2 in, 2 out]
              n279 = Greater Or Equal?(x=w262, y=w263) -> (x >= y?=w261:bool)
              n280 = local write "prep_done"(w261) -> ()
            }
            frame #2 {
              n281 = local read "run started"() -> (w265:bool)
              n282 = Not(x=w265) -> (.not. x?=w264:bool)
              n283 = stacked-sequence {
                tunnel: w264 -> [w267 w273 w282 w291 w300 w309 w318 w327]
                frame #0 {
                  n284 = case shown="True" w267 {
                    tunnel: ["run: " "pre-run: "] -> w266
                    frame False {
                    }
                    frame True {
                    }
                  }
                  n285 = property on="Status Out" class="Str"("Value"=w266) -> ()  [unwired: 2 in, 2 out]
                }
                frame #1 {
                  n286 = property on="Al bubbler" class="Clust (strict)"() -> ("Value"=w270:T7)  [unwired: 2 in, 2 out]
                  n287 = Unbundle By Name(w270) -> ("Run"=w272:bool, "Prep"=w271:bool)
                  n288 = property on="Status Out" class="Str"() -> ("Value"=w278:string)  [unwired: 2 in, 2 out]
                  n289 = call "flow_strings.vi"("string in"=w278, "is first in?"=TRUE, "name"="Al", "run source?"=w272, "prep source?"=w271, "is prep?"=w273) -> ("string out"=w277:string, "is first out?"=w276:bool)  [unwired: 1 in]
                  n290 = property on="Status Out" class="Str"("Value"=w277) -> ()  [unwired: 2 in, 2 out]
                  n291 = property on="first" class="Bool (strict)"("Value"=w276) -> ()  [unwired: 2 in, 2 out]
                }
                frame #2 {
                  n292 = property on="Ga bubbler" class="Clust (strict)"() -> ("Value"=w281:T8)  [unwired: 2 in, 2 out]
                  n293 = Unbundle By Name(w281) -> ("Bubbler (main).Run"=w280:bool, "Bubbler (main).Prep"=w279:bool)
                  n294 = property on="Status Out" class="Str"() -> ("Value"=w286:string)  [unwired: 2 in, 2 out]
                  n295 = property on="first" class="Bool (strict)"() -> ("Value"=w284:bool)  [unwired: 2 in, 2 out]
                  n296 = call "flow_strings.vi"("string in"=w286, "is first in?"=w284, "name"="Ga", "run source?"=w280, "prep source?"=w279, "is prep?"=w282) -> ("string out"=w287:string, "is first out?"=w283:bool)  [unwired: 1 in]
                  n297 = property on="Status Out" class="Str"("Value"=w287) -> ()  [unwired: 2 in, 2 out]
                  n298 = property on="first" class="Bool (strict)"("Value"=w283) -> ()  [unwired: 2 in, 2 out]
                }
                frame #3 {
                  n299 = property on="In bubbler" class="Clust (strict)"() -> ("Value"=w290:T7)  [unwired: 2 in, 2 out]
                  n300 = Unbundle By Name(w290) -> ("Run"=w289:bool, "Prep"=w288:bool)
                  n301 = property on="Status Out" class="Str"() -> ("Value"=w296:string)  [unwired: 2 in, 2 out]
                  n302 = property on="first" class="Bool (strict)"() -> ("Value"=w294:bool)  [unwired: 2 in, 2 out]
                  n303 = call "flow_strings.vi"("string in"=w296, "is first in?"=w294, "name"="In", "run source?"=w289, "prep source?"=w288, "is prep?"=w291) -> ("string out"=w293:string, "is first out?"=w292:bool)  [unwired: 1 in]
                  n304 = property on="Status Out" class="Str"("Value"=w293) -> ()  [unwired: 2 in, 2 out]
                  n305 = property on="first" class="Bool (strict)"("Value"=w292) -> ()  [unwired: 2 in, 2 out]
                }
                frame #4 {
                  n306 = property on="P gas" class="Clust (strict)"() -> ("Value"=w299:T7)  [unwired: 2 in, 2 out]
                  n307 = Unbundle By Name(w299) -> ("Run"=w298:bool, "Prep"=w297:bool)
                  n308 = property on="Status Out" class="Str"() -> ("Value"=w304:string)  [unwired: 2 in, 2 out]
                  n309 = property on="first" class="Bool (strict)"() -> ("Value"=w302:bool)  [unwired: 2 in, 2 out]
                  n310 = call "flow_strings.vi"("string in"=w304, "is first in?"=w302, "name"="PH3", "run source?"=w298, "prep source?"=w297, "is prep?"=w300) -> ("string out"=w303:string, "is first out?"=w301:bool)  [unwired: 1 in]
                  n311 = property on="Status Out" class="Str"("Value"=w303) -> ()  [unwired: 2 in, 2 out]
                  n312 = property on="first" class="Bool (strict)"("Value"=w301) -> ()  [unwired: 2 in, 2 out]
                }
                frame #5 {
                  n313 = property on="As gas" class="Clust (strict)"() -> ("Value"=w308:T7)  [unwired: 2 in, 2 out]
                  n314 = Unbundle By Name(w308) -> ("Run"=w307:bool, "Prep"=w306:bool)
                  n315 = property on="Status Out" class="Str"() -> ("Value"=w313:string)  [unwired: 2 in, 2 out]
                  n316 = property on="first" class="Bool (strict)"() -> ("Value"=w311:bool)  [unwired: 2 in, 2 out]
                  n317 = call "flow_strings.vi"("string in"=w313, "is first in?"=w311, "name"="AsH3", "run source?"=w307, "prep source?"=w306, "is prep?"=w309) -> ("string out"=w310:string, "is first out?"=w312:bool)  [unwired: 1 in]
                  n318 = property on="Status Out" class="Str"("Value"=w310) -> ()  [unwired: 2 in, 2 out]
                  n319 = property on="first" class="Bool (strict)"("Value"=w312) -> ()  [unwired: 2 in, 2 out]
                }
                frame #6 {
                  n320 = property on="P bubbler" class="Clust (strict)"() -> ("Value"=w317:T7)  [unwired: 2 in, 2 out]
                  n321 = Unbundle By Name(w317) -> ("Run"=w316:bool, "Prep"=w315:bool)
                  n322 = property on="Status Out" class="Str"() -> ("Value"=w323:string)  [unwired: 2 in, 2 out]
                  n323 = property on="first" class="Bool (strict)"() -> ("Value"=w321:bool)  [unwired: 2 in, 2 out]
                  n324 = call "flow_strings.vi"("string in"=w323, "is first in?"=w321, "name"="P liq", "run source?"=w316, "prep source?"=w315, "is prep?"=w318) -> ("string out"=w320:string, "is first out?"=w319:bool)  [unwired: 1 in]
                  n325 = property on="Status Out" class="Str"("Value"=w320) -> ()  [unwired: 2 in, 2 out]
                  n326 = property on="first" class="Bool (strict)"("Value"=w319) -> ()  [unwired: 2 in, 2 out]
                }
                frame #7 {
                  n327 = property on="Se bubbler" class="Clust (strict)"() -> ("Value"=w326:T8)  [unwired: 2 in, 2 out]
                  n328 = Unbundle By Name(w326) -> ("Bubbler (main).Run"=w325:bool, "Bubbler (main).Prep"=w324:bool)
                  n329 = property on="Status Out" class="Str"() -> ("Value"=w332:string)  [unwired: 2 in, 2 out]
                  n330 = property on="first" class="Bool (strict)"() -> ("Value"=w330:bool)  [unwired: 2 in, 2 out]
                  n331 = call "flow_strings.vi"("string in"=w332, "is first in?"=w330, "name"="Se", "run source?"=w325, "prep source?"=w324, "is prep?"=w327) -> ("string out"=w329:string, "is first out?"=w328:bool)  [unwired: 1 in]
                  n332 = property on="Status Out" class="Str"("Value"=w329) -> ()  [unwired: 2 in, 2 out]
                  n333 = property on="first" class="Bool (strict)"("Value"=w328) -> ()  [unwired: 2 in, 2 out]
                }
              }
            }
            frame #3 {
              n334 = property on="run started" class="Bool (strict)"() -> ("Value"=w338:bool)  [unwired: 2 in, 2 out]
              n335 = Not(x=w338) -> (.not. x?=w337:bool)
              n336 = property on="prep_done" class="Bool (strict)"() -> ("Value"=w339:bool)  [unwired: 2 in, 2 out]
              n337 = And(x=w339, y=w337) -> (x .and. y?=w333:bool)
              n338 = case shown="True" w333 {
                selector: w333 -> [_ w341]
                tunnel: w336 -> [w340 w344]
                tunnel: [w340 w343] -> w335
                tunnel: w334 -> [_ w342]
                frame False {
                }
                frame True {
                  n339 = stacked-sequence {
                    tunnel: w342 -> [w346 _]
                    tunnel: w344 -> [_ w356]
                    tunnel: [_ w355] -> w343
                    tunnel: w341 -> [w345 _]
                    frame #0 {
                      n340 = case shown="False" w346 {
                        tunnel: w345 -> [w354 _]
                        frame False {
                          n341 = property on="Ga bubbler" class="Clust (strict)"() -> ("Value"=w352:T8)  [unwired: 2 in, 2 out]
                          n342 = property on="In bubbler" class="Clust (strict)"() -> ("Value"=w351:T7)  [unwired: 2 in, 2 out]
                          n343 = property on="Se bubbler" class="Clust (strict)"() -> ("Value"=w347:T8)  [unwired: 2 in, 2 out]
                          n344 = property on="P gas" class="Clust (strict)"() -> ("Value"=w350:T7)  [unwired: 2 in, 2 out]
                          n345 = property on="Al bubbler" class="Clust (strict)"() -> ("Value"=w353:T7)  [unwired: 2 in, 2 out]
                          n346 = property on="As gas" class="Clust (strict)"() -> ("Value"=w349:T7)  [unwired: 2 in, 2 out]
                          n347 = property on="P bubbler" class="Clust (strict)"() -> ("Value"=w348:T7)  [unwired: 2 in, 2 out]
                          n348 = call "Set_V_III.vi"("Se bubbler"=w347, "P bubbler"=w348, "As gas"=w349, "P gas"=w350, "Run Started"=w354, "In bubbler"=w351, "Ga bubbler"=w352, "Al bubbler"=w353) -> ()  [unwired: 4 in]
                        }
                        frame True {
                        }
                      }
                    }
                    frame #1 {
                      n349 = call "Set_Argument.vi"("Enable"=TRUE, "Argument"="run_started", "Argument List In"=w356) -> ("Argument List Out"=w355:string[])
                    }
                  }
                }
              }
            }
          }
        }
        frame "End" {
        }
        frame "Idle" {
        }
      }
    }
  }
  "Argument List Out" <- w10
